vi "Engine_PreBuild.vi"(5 "New Job":T5, 7 "NewItem":T6, 8 "ErrIn":errorcluster, 10 "errorMsg":T1, 11 "MSI in":refnum<class "IB_MSI.lvclass">) -> (0 "ErrOut":errorcluster, 2 "InstallerFiles":T2[](array[typedef]) {"TargetType" items=["Relative to default installation directory"=68, "Root directory on first partition"=70, "Relative to directory table key"=82, "Absolute path to file"=65]}, 3 "MSI out":refnum<class "IB_MSI.lvclass">)   [LabVIEW 2020, in "IB_MSI.lvclass"]
uses:
  <vilib>/AppBuilder/IB_Classes/MSI/IB_MSI.lvclass
  <vilib>/AppBuilder/IB_Classes/MSI/IB_MSI.lvclass/IB_MSI.ctl
  <resource>/Framework/Providers/Builds/Installer/CDK_GLOBAL_STRINGS.vi
  <resource>/Framework/Providers/Builds/Installer/CDK_sTypeDef_DevPartShortcut.ctl
  <vilib>/AppBuilder/IB_Classes/Installer/Installer.lvclass
  <vilib>/AppBuilder/IB_Classes/Source/File/IB_Source_File.lvclass
  <vilib>/AppBuilder/IB_Classes/Source/IB_Source.lvclass
  <vilib>/AppBuilder/IB_Classes/Shortcut/IB_Shortcut.lvclass
  <vilib>/AppBuilder/IB_Classes/Destination/IB_Destination.lvclass
  <resource>/Framework/Providers/Builds/Installer/CDK_GLOBAL_LABELS.vi
  e:/builds/penguin/labview/branches/2020/dev/dist/vi.lib/AppBuilder/IB_Classes/Installer/Installer.lvclass
  e:/builds/penguin/labview/branches/2020/dev/dist/vi.lib/AppBuilder/IB_Classes/MSI/IB_MSI.lvclass
  e:/builds/penguin/labview/branches/2020/dev/dist/vi.lib/AppBuilder/IB_Classes/Source/IB_Source.lvclass
  e:/builds/penguin/labview/branches/2020/dev/dist/vi.lib/AppBuilder/IB_Classes/Source/File/IB_Source_File.lvclass
  <resource>/Framework/Providers/API/mxLvBuildNewItem.ctl
  <resource>/Framework/Providers/API/mxLvBuildNewJob.ctl
  <resource>/Framework/Providers/Builds/Installer/CDK_sTypeDef_DevPartInventory.ctl
  AppLibs/distkit/MDF/NIMdf.llb/MDFBDPAddFilePathType.ctl
  AppLibs/distkit/MDF/NI_MDF.lvlib
  <resource>/Framework/Providers/API/mxLvBuildError.ctl
panel:
  in  "dummy":T2={"Source"=path "", "FileTag"="", "RelPath"="", "Attributes"=0, "RegCOM"=FALSE, "TargetType"=68, "shortcuts"=[], "EXE_install"=FALSE, "EXE_uninstall"=FALSE, "unlock?"=FALSE, "CmdArg_install"="", "CmdArg_uninstall"=""} {"TargetType" items=["Relative to default installation directory"=68, "Root directory on first partition"=70, "Relative to directory table key"=82, "Absolute path to file"=65]}
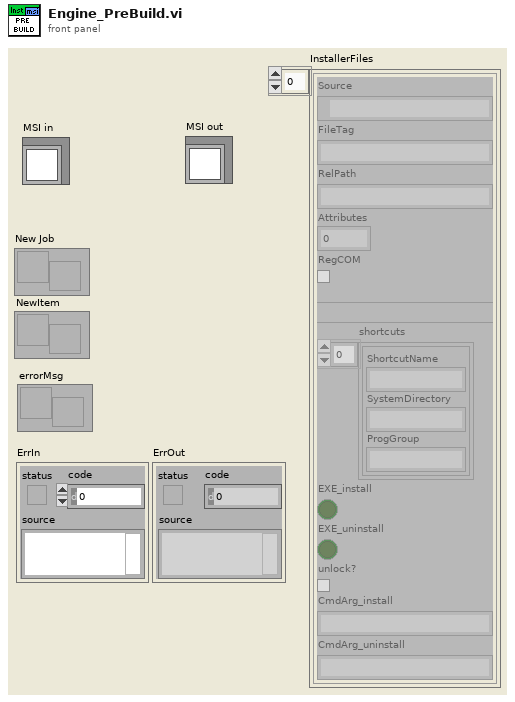
[diagram p1: front panel]
types:
  T1 = typedef "mxLvBuildError.ctl" = refnum<user-event>
  T2 = typedef "CDK_sTypeDef_DevPartInventory.ctl" = cluster{"Source":path, "FileTag":string, "RelPath":string, "Attributes":i32, "RegCOM":bool, "TargetType":T3, "shortcuts":T4[], "EXE_install":bool, "EXE_uninstall":bool, "unlock?":bool, "CmdArg_install":string, "CmdArg_uninstall":string}
  T3 = typedef "NI_MDF.lvlib/MDFBDPAddFilePathType.ctl" = i32
  T4 = typedef "CDK_sTypeDef_DevPartShortcut.ctl" = cluster{"ShortcutName":string, "SystemDirectory":string, "ProgGroup":string}
  T5 = typedef "mxLvBuildNewJob.ctl" = refnum<user-event>
  T6 = typedef "mxLvBuildNewItem.ctl" = refnum<user-event>
  T7 = typedef "CDK_sTypeDef_FileList.ctl" = cluster{"FileInventory":refnum<class "IB_Source_File.lvclass">, "containerID":string}
  T8 = typedef "IB_Installer.ctl" = cluster{"Destination":refnum<class "IB_Destination.lvclass">[], "Source":refnum<class "IB_Source.lvclass">[], "buildObject":T9, "defaultDir":string, "platform":string, "author":string, "productName":string, "buildSpecName":string, "hide":bool, "requireLVDevSys":bool, "autoIncrement":bool, "includeError":bool, "readmeID":string, "buildLocation":path, "readmePath":path, "mediaSize":u16, "language":T10, "productVersion":T11, "preview":bool, "programmatic":bool, "progressBarEvents":T12, "userLog_Path":path, "shortcutAddresses":T13[], "EXE_Install Address":string, "EXE_Uninstall Address":string, "additional NIPaths":refnum<class "Dest_NI_NIPath.lvclass">[], "web service itemIDs":string[], "installerName":string}
  T9 = typedef "ItemRef.ctl" = u64
  T10 = typedef "CDK_sTypeDef_Languages.ctl" = u16
  T11 = typedef "CDK_sTypeDef_ProductVersion.ctl" = cluster{"Major":u8, "Minor":u8, "Update":u16}
  T12 = typedef "provcom_ProgressBar_Events.ctl" = cluster{"newJob":refnum<user-event>, "newItem":refnum<user-event>, "errorMsg":T1, "cancel":refnum<user-event>}
  T13 = typedef "CDK_sTypeDef_ShortcutAddress.ctl" = cluster{"file":string, "shortcut":string}
  T14 = typedef "IB_Source.ctl" = cluster{"name":string, "sourceTag":string, "destTag":string, "path":path, "eng_installPath":string, "UI_inBuild?":bool, "str ref?":bool}
  T15 = typedef "IB_Source_File.ctl" = cluster{"Attributes":i16, "RegCOM":bool, "unlock":bool, "shortcuts":refnum<class "IB_Shortcut.lvclass">[], "EXE_install":bool, "CmdArg_install":string, "EXE_uninstall":bool, "CmdArg_uninstall":string}
  T16 = typedef "IB_Shortcut.ctl" = cluster{"name":string, "destIndex":i32, "subDir":string, "address":string}
  T17 = typedef "IB_Destination.ctl" = cluster{"name":string, "unlock":bool, "parentTag":string, "destTag":string, "eng_installPath":string}
  T18 = typedef "IB_MSI.ctl" = cluster{"upgradeCode":string, "distID":string, "windowMessage":string, "windowTitle":string, "arpPhone":string, "arpContact":string, "arpURL":string, "arpCompany":string, "licenseID":string, "licensePath":path, "welcomeImageID":string, "welcomeImagePath":path, "bannerImageID":string, "bannerImagePath":path, "osCheck":i32, "msiFileName":string, "cabFileName":string, "hwOption":T19, "hwPath":path, "regGroup":refnum<class "IB_RegGroup.lvclass">[], "regDest":refnum<class "IB_RegDest.lvclass">[], "selectedDists":refnum<class "IB_DistPart.lvclass">[], "installedDists":refnum<class "IB_DistPart.lvclass">[], "postInstallSteps":refnum<class "IB_Post_Install_Step.lvclass">[], "preUninstallSteps":refnum<class "IB_Post_Install_Step.lvclass">[], "winsec.certificate":string, "winsec.timestamp":string, "winsec.description":string, "autoselect drivers":bool, "hide non-runtimes":bool}
  T19 = typedef "CDK_sTypeDef_HWImportOption.ctl" = enum16{"<none>", "Merge", "Replace", "Dialog"}
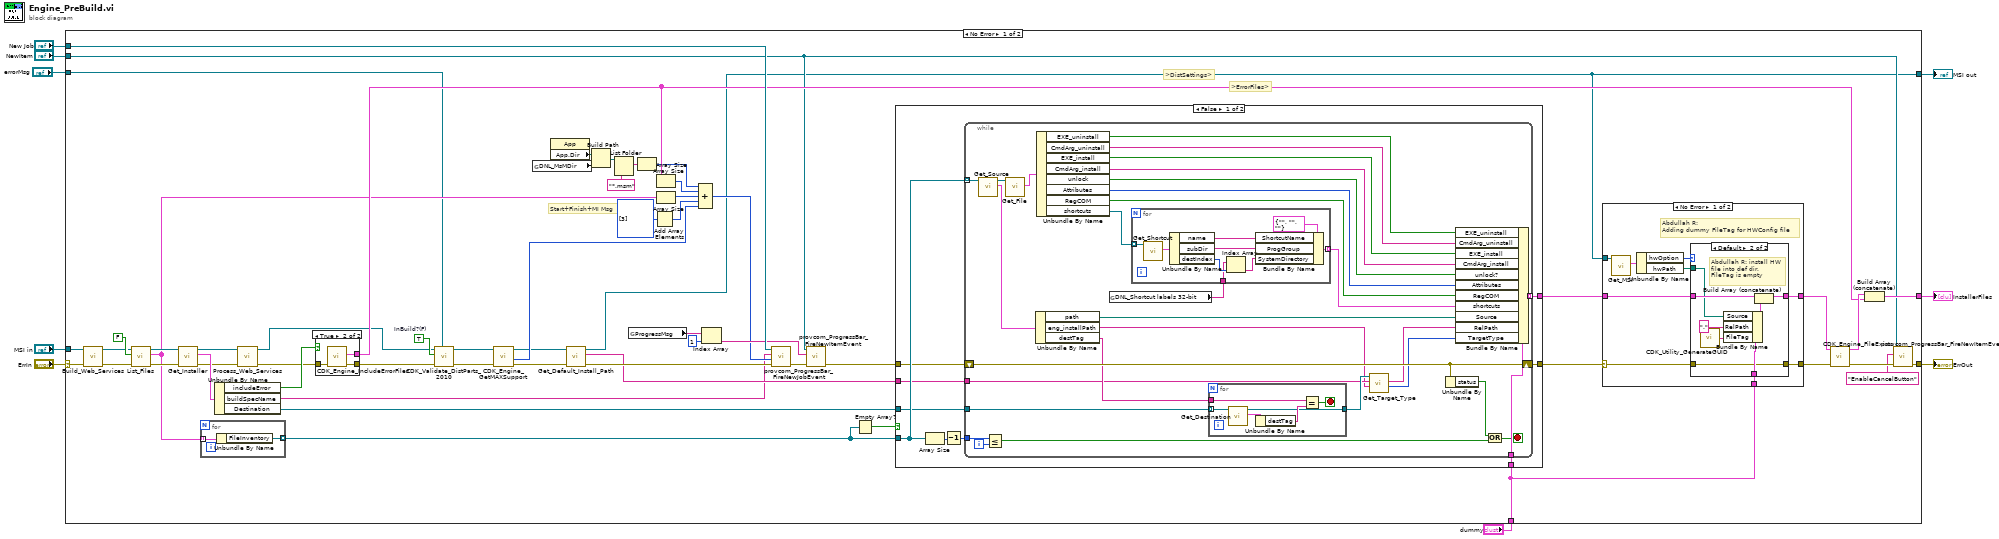
[diagram p0: block diagram]
diagram:
  n1 = case shown="No Error" "ErrIn" {
    selector: "ErrIn" -> [w13 w151]
    tunnel: [w41 w151] -> w8
    tunnel: "New Job" -> [w66 _]
    tunnel: "NewItem" -> [w39 _]
    tunnel: [w56 _] -> w5
    tunnel: "dummy" -> [w58 _]
    tunnel: [w23 w150] -> w3
    tunnel: "MSI in" -> [w15 w150]
    tunnel: "errorMsg" -> [w10 _]
    frame No Error {
      w31 = TRUE  # InBuild?(F)
      # ">DistSettings>"
      # ">ErrorFiles>"
      # "Start+Finish+MI Msg"
      n2 = call <vilib>:"Build_Web_Services.vi"("error in (no error)"=w13, "Installer in"=w15) -> ("error out"=w12:errorcluster, "Installer out"=w14:refnum<class "IB_MSI.lvclass">)  [unwired: 8 in]
      n3 = call <vilib>:"List_Files.vi"("error in (no error)"=w12, "include unused? (T)"=FALSE, "Installer in"=w14) -> ("error out"=w33:errorcluster, "files"=w30:T7[], "Installer out"=w32:refnum<class "IB_MSI.lvclass">)  [unwired: 6 out]
      n4 = call <vilib>:"Get_Installer.vi"("error in (no error)"=w33, "Installer in"=w32) -> ("error out"=w22:errorcluster, "data"=w38:T8, "Installer out"=w20:refnum<class "IB_MSI.lvclass">)  [unwired: 7 out]
      n5 = for {
        tunnel: w30 -> [w69] mode=indexing
        tunnel: [w68] -> w29 mode=indexing
        n6 = Unbundle By Name(w69) -> ("FileInventory"=w68:refnum<class "IB_Source_File.lvclass">)
      }
      n7 = Unbundle By Name(w38) -> ("includeError"=w37:bool, "buildSpecName"=w16:string, "Destination"=w28:refnum<class "IB_Destination.lvclass">[])
      n8 = call <vilib>:"Process_Web_Services.vi"("error in (no error)"=w22, "IB_MSI in"=w20) -> ("error out"=w21:errorcluster, "IB_MSI out"=w19:refnum<class "IB_MSI.lvclass">)  [unwired: 8 out]
      n9 = case shown="True" w37 {
        tunnel: [w70 w73] -> w34
        tunnel: [_ w72] -> w54
        tunnel: w21 -> [w70 w71]
        frame False {
        }
        frame True {
          n10 = call <resource>:"CDK_Engine_IncludeErrorFiles.vi"("ErrIn"=w71) -> ("ErrOut"=w73:errorcluster, "ErrorFiles"=w72:T2[])  [unwired: 1 in, 8 out]
        }
      }
      n11 = call <resource>:"CDK_Validate_DistParts_2010.vi"("errorMsg"=w10, "ErrIn"=w34, "InBuild(F)"=w31, "IB_MSI.lvclass"=w19) -> ("ErrOut"=w11:errorcluster, "IB_MSI.lvclass out"=w36:refnum<class "IB_MSI.lvclass">)  [unwired: 1 in, 5 out]
      n12 = call <resource>:"CDK_Engine_GetMAXSupport.vi"("IB_MSI.lvclass"=w36, "ErrIn"=w11) -> ("IB_MSI.lvclass out"=w24:refnum<class "IB_MSI.lvclass">, "ProdInfoSize"=w50:i32, "ErrOut"=w27:errorcluster)  [unwired: 3 in, 3 out]
      n13 = global read "CDK_GLOBAL_STRINGS.vi" "DNL_MsMDir"() -> (w46:path)
      n14 = property class="App"() -> ("App.Dir"=w45:path)  [unwired: 2 in, 2 out]
      n15 = call <vilib>:"Get_Default_Install_Path.vi"("error in (no error)"=w27, "Installer in"=w24) -> ("error out"=w26:errorcluster, "default_installPath"=w25:string, "Installer out"=w23:refnum<class "IB_MSI.lvclass">)  [unwired: 7 out]
      n16 = Build Path(base path=w45, name or relative path=w46) -> (appended path=w48:path)
      n17 = List Folder(path=w48, pattern="*.msm") -> (filenames=w49:string[])  [unwired: 1 in, 4 out]
      n18 = global read "CDK_GLOBAL_STRINGS.vi" "ProgressMsg"() -> (w65:string[])
      n19 = Array Size(array=w49) -> (size(s)=w44:i32)
      n20 = Add Array Elements(numeric array=i32[] [3]) -> (sum=w63:i32)
      n21 = Array Size(array=w54) -> (size(s)=w62:i32)
      n22 = Array Size(array=w30) -> (size(s)=w61:i32)
      n23 = Compound Arithmetic op=ADD(w44, w62, w61, w63, w50) -> (w60:i32)
      n24 = Index Array(array=w65, index=1) -> (element=w64:string)
      n25 = call <resource>:"provcom_ProgressBar_FireNewJobEvent.vi"("error in (no error)"=w26, "#ofItems"=w60, "Label"=w16, "New Job"=w66) -> ("error out"=w43:errorcluster)  [unwired: 7 out]
      n26 = call <resource>:"provcom_ProgressBar_FireNewItemEvent.vi"("error in (no error)"=w43, "Label"=w64, "NewItem"=w39) -> ("error out"=w35:errorcluster)  [unwired: 8 out]
      n27 = Empty Array?(array=w29) -> (empty?=w59:bool)
      n28 = case shown="False" w59 {
        tunnel: w58 -> [w82 _]
        tunnel: [w78 w128] -> w51
        tunnel: w35 -> [w75 w128]
        tunnel: w25 -> [w76 _]
        tunnel: w29 -> [w79 _]
        tunnel: [w77 _] -> w52
        tunnel: w28 -> [w74 _]
        frame False {
          n29 = Array Size(array=w79) -> (size(s)=w81:i32)
          n30 = Decrement(x=w81) -> (x-1=w80:i32)
          n31 = while {
            tunnel: w79 -> [w102] mode=indexing
            tunnel: w82 -> [w112]
            shift-right: [w95] -> w78
            shift-left: w75 -> [w95]
            tunnel: [w109] -> w77 mode=indexing
            tunnel: w80 -> [w107]
            tunnel: w76 -> [w89]
            tunnel: w74 -> [w94]
            i -> [w108]
            stop <- w104 stop-if-true
            n32 = call <vilib>:"Get_Source.vi"("IB_Source in"=w102) -> ("data"=w100:T14, "IB_Source out"=w101:refnum<class "IB_Source_File.lvclass">)  [unwired: 1 in, 8 out]
            n33 = Less Or Equal?(x=w107, y=w108) -> (x <= y?=w105:bool)
            n34 = call <vilib>:"Get_File.vi"("IB_Source_File in"=w101) -> ("data"=w103:T15)  [unwired: 1 in, 9 out]
            n35 = Unbundle By Name(w100) -> ("path"=w97:path, "eng_installPath"=w88:string, "destTag"=w93:string)
            n36 = Unbundle By Name(w103) -> ("EXE_uninstall"=w84:bool, "CmdArg_uninstall"=w83:string, "EXE_install"=w87:bool, "CmdArg_install"=w86:string, "unlock"=w96:bool, "Attributes"=w111:i16, "RegCOM"=w110:bool, "shortcuts"=w99:refnum<class "IB_Shortcut.lvclass">[])
            n37 = global read "CDK_GLOBAL_LABELS.vi" "DNL_Shortcut labels 32-bit"() -> (w85:string[])
            n38 = for {
              tunnel: w99 -> [w127] mode=indexing
              tunnel: [w124] -> w98 mode=indexing
              tunnel: w85 -> [w120]
              n39 = call <vilib>:"Get_Shortcut.vi"("Class in"=w127) -> ("data"=w126:T16)  [unwired: 1 in, 9 out]
              n40 = Unbundle By Name(w126) -> ("name"=w123:string, "subDir"=w122:string, "destIndex"=w121:i32)
              n41 = Index Array(array=w120, index=w121) -> (element=w119:string)
              n42 = Bundle By Name(cluster=T4 {"ShortcutName"="", "SystemDirectory"="", "ProgGroup"=""} ("CDK_sTypeDef_DevPartShortcut"), "ShortcutName"=w123, "ProgGroup"=w122, "SystemDirectory"=w119) -> (w124:T4)
            }
            n43 = for {
              tunnel: w94 -> [w118] mode=indexing
              tunnel: w93 -> [w116]
              tunnel: [w113] -> w92
              stop <- w114 stop-if-true
              n44 = call <vilib>:"Get_Destination.vi"("IB_Destination in"=w118) -> ("data"=w117:T17, "IB_Destination out"=w113:refnum<class "IB_Destination.lvclass">)  [unwired: 1 in, 8 out]
              n45 = Unbundle By Name(w117) -> ("destTag"=w115:string)
              n46 = Equal?(x=w116, y=w115) -> (x = y?=w114:bool)
            }
            n47 = call-dynamic "Get_Target_Type.vi"("install path"=w88, "default install path"=w89, "IB_Destination in"=w92) -> ("path for target type"=w90:T3, "path for target"=w91:string)  [unwired: 1 in, 6 out]
            n48 = Unbundle By Name(w95) -> ("status"=w106:bool)
            n49 = Bundle By Name(cluster=w112, "EXE_uninstall"=w84, "CmdArg_uninstall"=w83, "EXE_install"=w87, "CmdArg_install"=w86, "unlock?"=w96, "Attributes"=w111, "RegCOM"=w110, "shortcuts"=w98, "Source"=w97, "RelPath"=w91, "TargetType"=w90) -> (w109:T2)
            n50 = Or(x=w106, y=w105) -> (x .or. y?=w104:bool)
          }
        }
        frame True {
          # "Abdullah R:\nThis is no error. We are allowing empty installer\nthat may or may not have error files."
        }
      }
      n51 = case shown="No Error" w51 {
        selector: w51 -> [w133 w148]
        tunnel: w52 -> [w135 w149]
        tunnel: w58 -> [w134 _]
        tunnel: [w131 w149] -> w53
        tunnel: [w132 w148] -> w57
        tunnel: w23 -> [w129 _]
        frame No Error {
          # "Abdullah R:\nAdding dummy FileTag for HWConfig file"
          n52 = call <vilib>:"Get_MSI.vi"("IB_MSI in"=w129) -> ("data"=w130:T18)  [unwired: 1 in, 9 out]
          n53 = Unbundle By Name(w130) -> ("hwOption"=w137:T19, "hwPath"=w136:path)
          n54 = case shown="Default" w137 {
            tunnel: w133 -> [w138 w144]
            tunnel: w136 -> [_ w143]
            tunnel: w135 -> [w139 w147]
            tunnel: w134 -> [_ w146]
            tunnel: [w138 w144] -> w132
            tunnel: [w139 w141] -> w131
            frame "<none>" {
            }
            frame Default {
              # "Abdullah R: install HW\nfile into def dir.\nFileTag is empty"
              n55 = call <resource>:"CDK_Utility_GenerateGUID.vi"() -> ("GUID"=w140:string)  [unwired: 9 out]
              n56 = Bundle By Name(cluster=w146, "Source"=w143, "RelPath"=".", "FileTag"=w140) -> (w145:T2)
              n57 = Build Array (concatenate)(w147, w145) -> (w141:T2[])
            }
          }
        }
        frame Error {
        }
      }
      n58 = call <resource>:"CDK_Engine_FileExists.vi"("ErrIn"=w57, "InstallerFiles"=w53) -> ("ErrOut"=w42:errorcluster, "InstFiles"=w55:T2[])  [unwired: 8 out]
      n59 = Build Array (concatenate)(w55, w54) -> (w56:T2[])
      n60 = call <resource>:"provcom_ProgressBar_FireNewItemEvent.vi"("error in (no error)"=w42, "Label"="EnableCancelButton" ("element"), "NewItem"=w39) -> ("error out"=w41:errorcluster)  [unwired: 8 out]
    }
    frame Error {
    }
  }
  "ErrOut" <- w8
  "InstallerFiles" <- w5
  "MSI out" <- w3
